vi "Control Panel Initialization.vi"() -> (1 "ArmRotatedPicture":T1, 3 "ControlPanelRotatedPicture":T1)   [LabVIEW 2019]
doc: "Perform one time initialization for simulation."
uses:
  Rotated_Picture_TypeDef.ctl
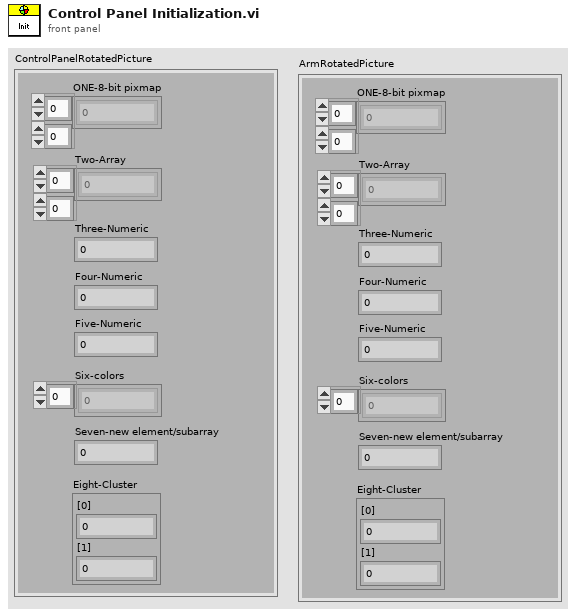
[diagram p1: front panel]
types:
  T1 = typedef "Rotated_Picture_TypeDef.ctl" = cluster{"ONE-8-bit pixmap":u8[][], "Two-Array":cdb[][], "Three-Numeric":i32, "Four-Numeric":i32, "Five-Numeric":cdb, "Six-colors":u32[], "Seven-new element/subarray":u32, "Eight-Cluster":cluster{"[0]":i32, "[1]":i32}}
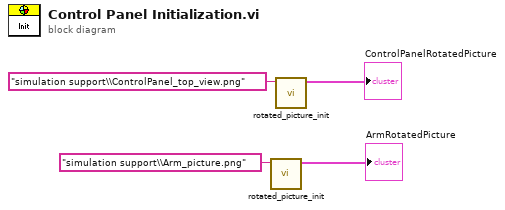
[diagram p0: block diagram]
diagram:
  n1 = call "rotated_picture_init.vi"("Picture FIle Name"="simulation support\\Arm_picture.png") -> ("RotatedPictureInfo"=→"ArmRotatedPicture":T1)  [unwired: 10 in]
  n2 = call "rotated_picture_init.vi"("Picture FIle Name"="simulation support\\ControlPanel_top_view.png") -> ("RotatedPictureInfo"=→"ControlPanelRotatedPicture":T1)  [unwired: 10 in]
